vi "_PC_DataChrom_Conv_CorrMS.vi"(5 "RepeatTimes_Input":u16[](array[numeric]), 7 "Y":dbl[](array[numeric]), 9 "X":dbl[](array[numeric])) -> (1 "Spectrum Y":dbl[](array[numeric]), 3 "Spectrum X":dbl[](array[numeric]), 4 "RepeatTimes_Output":u16[](array[numeric]))   [LabVIEW 2018]
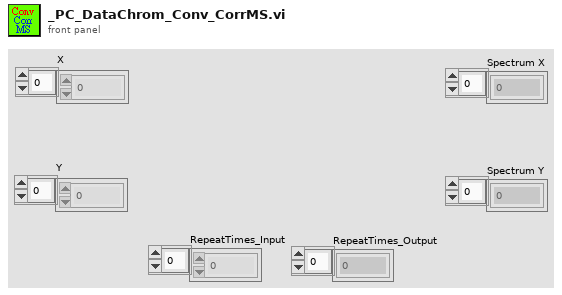
[diagram p1: front panel]
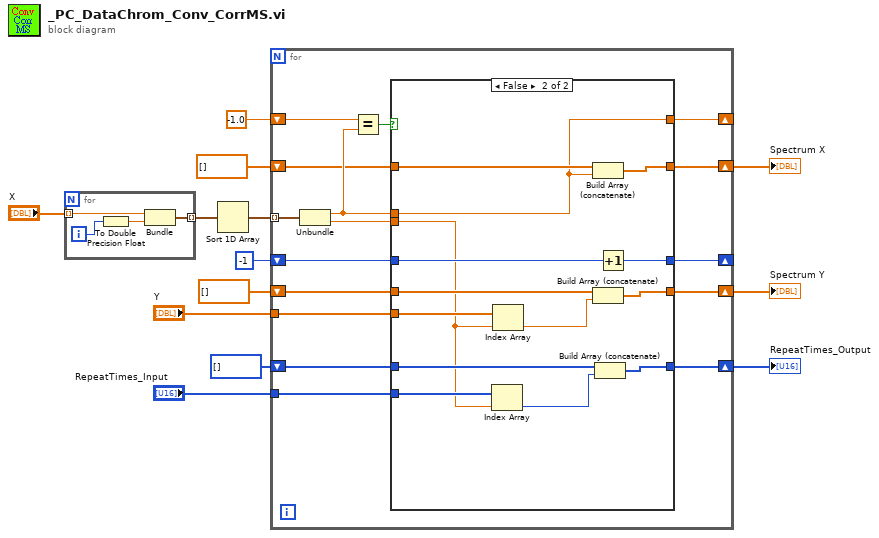
[diagram p0: block diagram]
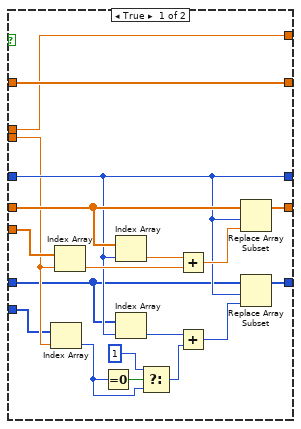
[diagram p2: hidden frame]
diagram:
  n1 = for {
    tunnel: "X" -> [w17] mode=indexing
    tunnel: [w14] -> w13 mode=indexing
    i -> [w16]
    n2 = To Double Precision Float(number=w16) -> (double precision float=w15:dbl)
    n3 = Bundle("Numeric"=w17, w15) -> (w14:cluster{"Numeric":dbl, dbl})  [unwired: 1 in]
  }
  n4 = Sort 1D Array(array=w13) -> (sorted array=w12:cluster{"Numeric":dbl, dbl}[])
  n5 = for {
    tunnel: w12 -> [w33] mode=indexing
    shift-right: [w27] -> _
    shift-left: -1.0 -> [w32]
    tunnel: "Y" -> [w29]
    shift-right: [w25] -> w6
    shift-left: dbl[] [] -> [w26]
    shift-right: [w22] -> _
    shift-left: -1 -> [w23]
    shift-right: [w21] -> w5
    shift-left: u16[] [] -> [w24]
    shift-right: [w19] -> w7
    shift-left: dbl[] [] -> [w20]
    tunnel: "RepeatTimes_Input" -> [w18]
    n6 = Unbundle(w33) -> ("Numeric"=w28:dbl, w30:dbl)
    n7 = Equal?(x=w32, y=w28) -> (x = y?=w31:bool)
    n8 = case shown="False" w31 {
      tunnel: w30 -> [w42 w54]
      tunnel: w29 -> [w51 w58]
      tunnel: w28 -> [w43 w60]
      tunnel: [w43 w60] -> w27
      tunnel: [w46 w56] -> w25
      tunnel: w26 -> [w50 w66]
      tunnel: w24 -> [w40 w63]
      tunnel: w23 -> [w44 w65]
      tunnel: [w44 w64] -> w22
      tunnel: [w45 w62] -> w21
      tunnel: w20 -> [w52 w61]
      tunnel: [w52 w59] -> w19
      tunnel: w18 -> [w41 w55]
      frame True {
        n9 = Index Array(array=w41, index=w42) -> (element=w35:u16)
        n10 = Index Array(array=w51, index=w42) -> (element=w48:dbl)
        n11 = Equal To 0?(x=w35) -> (x = 0?=w37:bool)
        n12 = Index Array(array=w50, index=w44) -> (element=w49:dbl)
        n13 = Index Array(array=w40, index=w44) -> (element=w39:u16)
        n14 = Select(t=u16 1, s=w37, f=w35) -> (s? t:f=w36:u16)
        n15 = Add(x=w49, y=w48) -> (x+y=w47:dbl)
        n16 = Add(x=w39, y=w36) -> (x+y=w38:u16)
        n17 = Replace Array Subset(array=w50, new element=w47, index=w44) -> (w46:dbl[])
        n18 = Replace Array Subset(array=w40, new element=w38, index=w44) -> (w45:u16[])
      }
      frame False {
        n19 = Index Array(array=w55, index=w54) -> (element=w53:u16)
        n20 = Index Array(array=w58, index=w54) -> (element=w57:dbl)
        n21 = Build Array (concatenate)(w61, w60) -> (w59:dbl[])
        n22 = Build Array (concatenate)(w66, w57) -> (w56:dbl[])
        n23 = Build Array (concatenate)(w63, w53) -> (w62:u16[])
        n24 = Increment(x=w65) -> (x+1=w64:i32)
      }
    }
  }
  "Spectrum X" <- w7
  "Spectrum Y" <- w6
  "RepeatTimes_Output" <- w5
